vi "Initialize with Topology (Device).vi"(8 "error in (no error)":errorcluster, 9 "reset device":bool=TRUE, 10 "topology":string, 11 "device":refnum<k21>) -> (0 "error out":errorcluster, 3 "session out":T1)   [LabVIEW 2020, in "SLSC Switch.lvlib"]
doc: "Returns a session handle used to identify the SLSC Switch module in all subsequent driver calls and sets the topology of the switch module."
uses:
  <vilib>/SLSC_Switch/SLSC Switch.lvlib
  nislscsl.dll
  <vilib>/userdefined/High Color/SLSC_Switch/nislscslSession.ctl
panel:
  in  "session in":T1
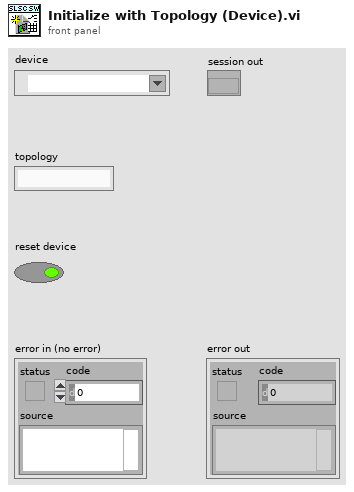
[diagram p1: front panel]
types:
  T1 = typedef "nislscslSession.ctl" = refnum<k20>
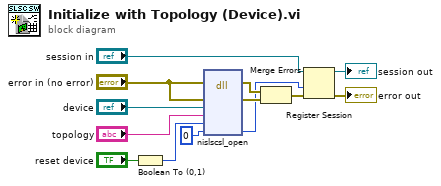
[diagram p0: block diagram]
diagram:
  n1 = Boolean To (0,1)(Boolean="reset device") -> (0, 1=w2:i16)
  n2 = dll-call lib="nislscsl.*" fn="nislscsl_open"(error in="error in (no error)", "errorCluster"="error in (no error)", "deviceIdentifier"="device", "topologyName"="topology", "reset"=w2, "sessionHandlePtr"=u64 0) -> (error out=w10:errorcluster, "errorCluster"=w9:errorcluster, "sessionHandlePtr"=w8:u64)  [unwired: 6 in, 1 out]
  n3 = Merge Errors(w10, w9) -> (w7:errorcluster)
  n4 = Register Session(8:w7, 9:w8, 11:"session in") -> (0:→"error out":errorcluster, 3:→"session out":T1)  [unwired: 2 in]
